vi "TTA_MATLAB_TxOutputPowerTest.vi"(0 "Sub-Function Name":string, 1 "Instrument Cluster In":T2, 5 "Test Group":string, 11 "error in":errorcluster) -> (4 "SubTestSuccess":dbl[](array[numeric]), 12 "Instrument Cluster Out":T2, 15 "error out":errorcluster)   [LabVIEW 2016]
uses:
  TTA_Controls/TTA_Control_Complete_Settings_Cluster.ctl
  TTA_Controls/TTA_Control_Instrument_Cluster.ctl
  TTA_Globals/TTA_Global_Complete_Settings.vi
panel:
  out "Tx Output \nPower Results":T1(array[cluster])
  out "Channel":string
  out "Tx":string
  out "Test Status":string
  in  "Complete Settings Cluster":T3
  out "RFICs":i32[](array[numeric])
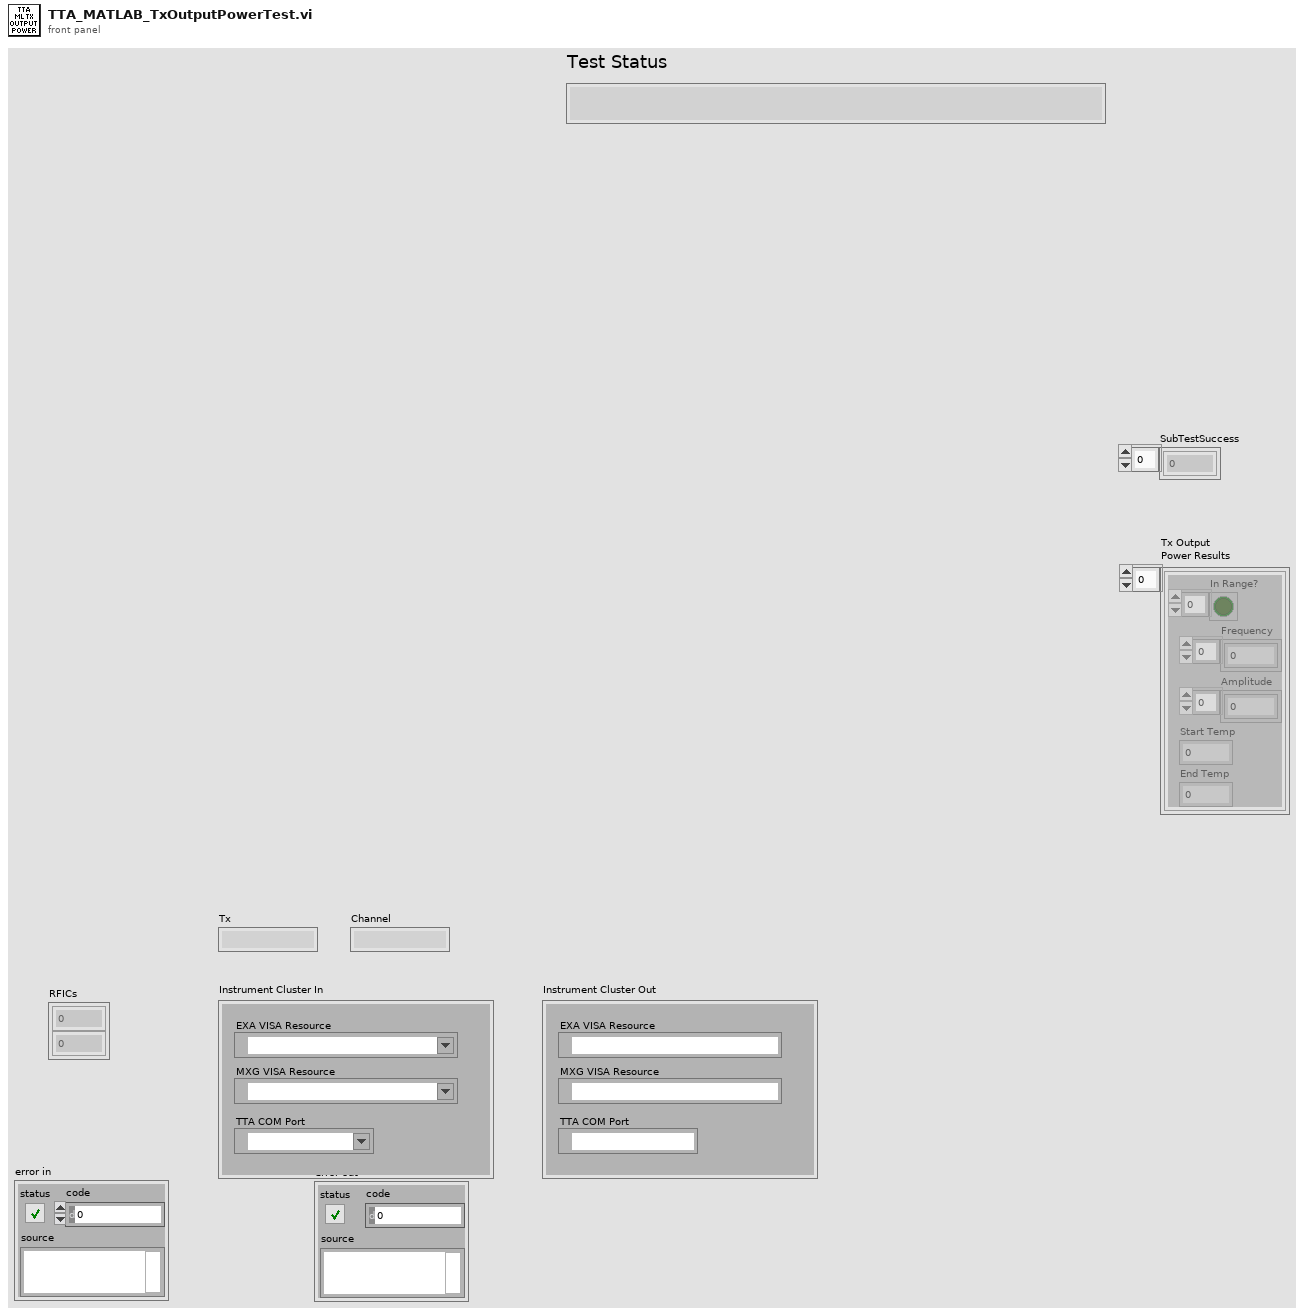
[diagram p1: front panel]
types:
  T1 = cluster{"In Range?":bool[], "Frequency":dbl[], "Amplitude":dbl[], "Start Temp":dbl, "End Temp":dbl}[]
  T2 = typedef "TTA_Control_Instrument_Cluster.ctl" = cluster{"EXA VISA Resource":refnum<visa-resource-name>, "MXG VISA Resource":refnum<visa-resource-name>, "TTA COM Port":refnum<visa-resource-name>}
  T3 = typedef "TTA_Control_Complete_Settings_Cluster.ctl" = cluster{"Brief Cluster":cluster{"STM Firmware File":string, "STM Firmware Address":string, "Required SW Version":string, "Template Used":string}, "Instrument Setting Cluster":cluster{"BDSFreq":dbl, "BDS Amp":dbl, "TxRFCal_Freq":dbl, "TxRFCal_Amp":dbl, "RxRFCal_Freq":dbl, "RxRFCal_Freq":dbl, "TxIF_Freq":dbl, "TxIF_Amp":dbl, "Tx_Output_Power_Signal_Freq":dbl, "Tx_ACPR_Signal_Freq":dbl, "Rx_RF_Freq":dbl, "Rx_RF_Amp":dbl, "Rx_Output_Power_Signal_Freq":dbl, "Rx_Output_Power_Sense_Freq":dbl}, "PAL Calibration\nInputs Cluster":cluster{"Amplitude Range\nMax(dBm)":dbl, "Amplitude Range\nMin(dBm)":dbl, "Amplitude Least\nCriteria (dBm)":dbl, "Frequency 1":dbl, "Frequency 2":dbl, "Frequency 3":dbl, "CAL Amplitude\nDecrement (dB)":dbl, "CAL Amplitude\nIncrement(dB)":dbl, "DownloadFile":string}, "TxOffset Cal Cluster":cluster{"Tx1 Offset (dB)":dbl, "Tx2 Offset (dB)":dbl, "Tx3 Offset (dB)":dbl, "Tx4 Offset (dB)":dbl, "Total RF Tx Loss (dB)":dbl}, "RxOffset Cal Cluster":cluster{"Rx1 Offset (dB)":dbl, "Rx2 Offset (dB)":dbl, "Rx3 Offset (dB)":dbl, "Rx4 Offset (dB)":dbl, "Total RF Rx Loss (dB)":dbl}, "TX Output Power Settings Cluster":cluster{"Frequency Sweep (MHz)":dbl[], "Sig Gen \nPower (dBm)":dbl, "Span (kHz)":dbl, "RBW (Hz)":dbl, "Ref Level (dBm)":dbl, "Low Power \nLimit":dbl, "High Power \nLimit":dbl, "DigAtt Max":dbl, "DigAtt Min":dbl}, "Tx ACPR Settings Cluster":cluster{"ACPR Filename":string, "Sampling Rate":dbl, "Power (dBm)":dbl, "IF Frequency Sweep (MHz)":dbl[], "State Name":string, "Mechanical\nAttenuation":dbl, "RefLevel Offset":dbl, "Amplitude Range\nMax (dBm)":dbl, "Amplitude Range\nMin (dBm)":dbl, "Cal Amp \nIncrement (dB)":dbl, "Cal Amp\nDecrement (dB)":dbl}, "Power Cal Cluster":cluster{"Power List (dBm)":dbl[], "Frequency (MHz)":dbl[], "Cal Decrement (dB)":dbl, "Cal Increment (dB)":dbl}, "Rx Received Power Settings Cluster":cluster{"Frequency Sweep (MHz)":dbl[], "Power (dBm)":dbl, "Span (kHz)":dbl, "RBW (Hz)":dbl, "Ref Level":dbl, "Low Power \nLimit (dBm)":dbl, "High Power\nLimit (dBm)":dbl}, "Tx Output Power Criteria Cluster":cluster{"CH1-TX1 \nMin":dbl, "CH1-TX1\nMax":dbl, "CH1-TXx3\nMin ":dbl, "CH1-TXx3\nMax":dbl, "CH2-TX1\nMin":dbl, "CH2-TX1\nMax":dbl, "CH2-TXx3\nMin":dbl, "CH2-TXx3\nMax":dbl}, "Tx ACPR Criteria Cluster":cluster{"Min Inband":dbl, "Max Close Outband":dbl, "Max Far Outband":dbl}, "Rx Output Power Criteria Cluster":cluster{"CH1-RX1 \nMin":dbl, "CH1-RX1 \nMax":dbl, "CH1-RXx3 \nMin":dbl, "CH1-RXx3\nMax":dbl, "CH2-RX1\nMin":dbl, "CH2-RX1\nMax":dbl, "CH2-RXx3\nMin":dbl, "CH2-RXx3\nMax":dbl}}
  T4 = cluster{"Amplitude Range\nMax(dBm)":dbl, "Amplitude Range\nMin(dBm)":dbl, "Amplitude Least\nCriteria (dBm)":dbl, "Frequency 1":dbl, "Frequency 2":dbl, "Frequency 3":dbl, "CAL Amplitude\nDecrement (dB)":dbl, "CAL Amplitude\nIncrement(dB)":dbl, "DownloadFile":string}
  T5 = cluster{"Frequency Sweep (MHz)":dbl[], "Sig Gen \nPower (dBm)":dbl, "Span (kHz)":dbl, "RBW (Hz)":dbl, "Ref Level (dBm)":dbl, "Low Power \nLimit":dbl, "High Power \nLimit":dbl, "DigAtt Max":dbl, "DigAtt Min":dbl}
  T6 = cluster{"In Range?":bool[], "Frequency":dbl[], "Amplitude":dbl[], "Start Temp":dbl, "End Temp":dbl}
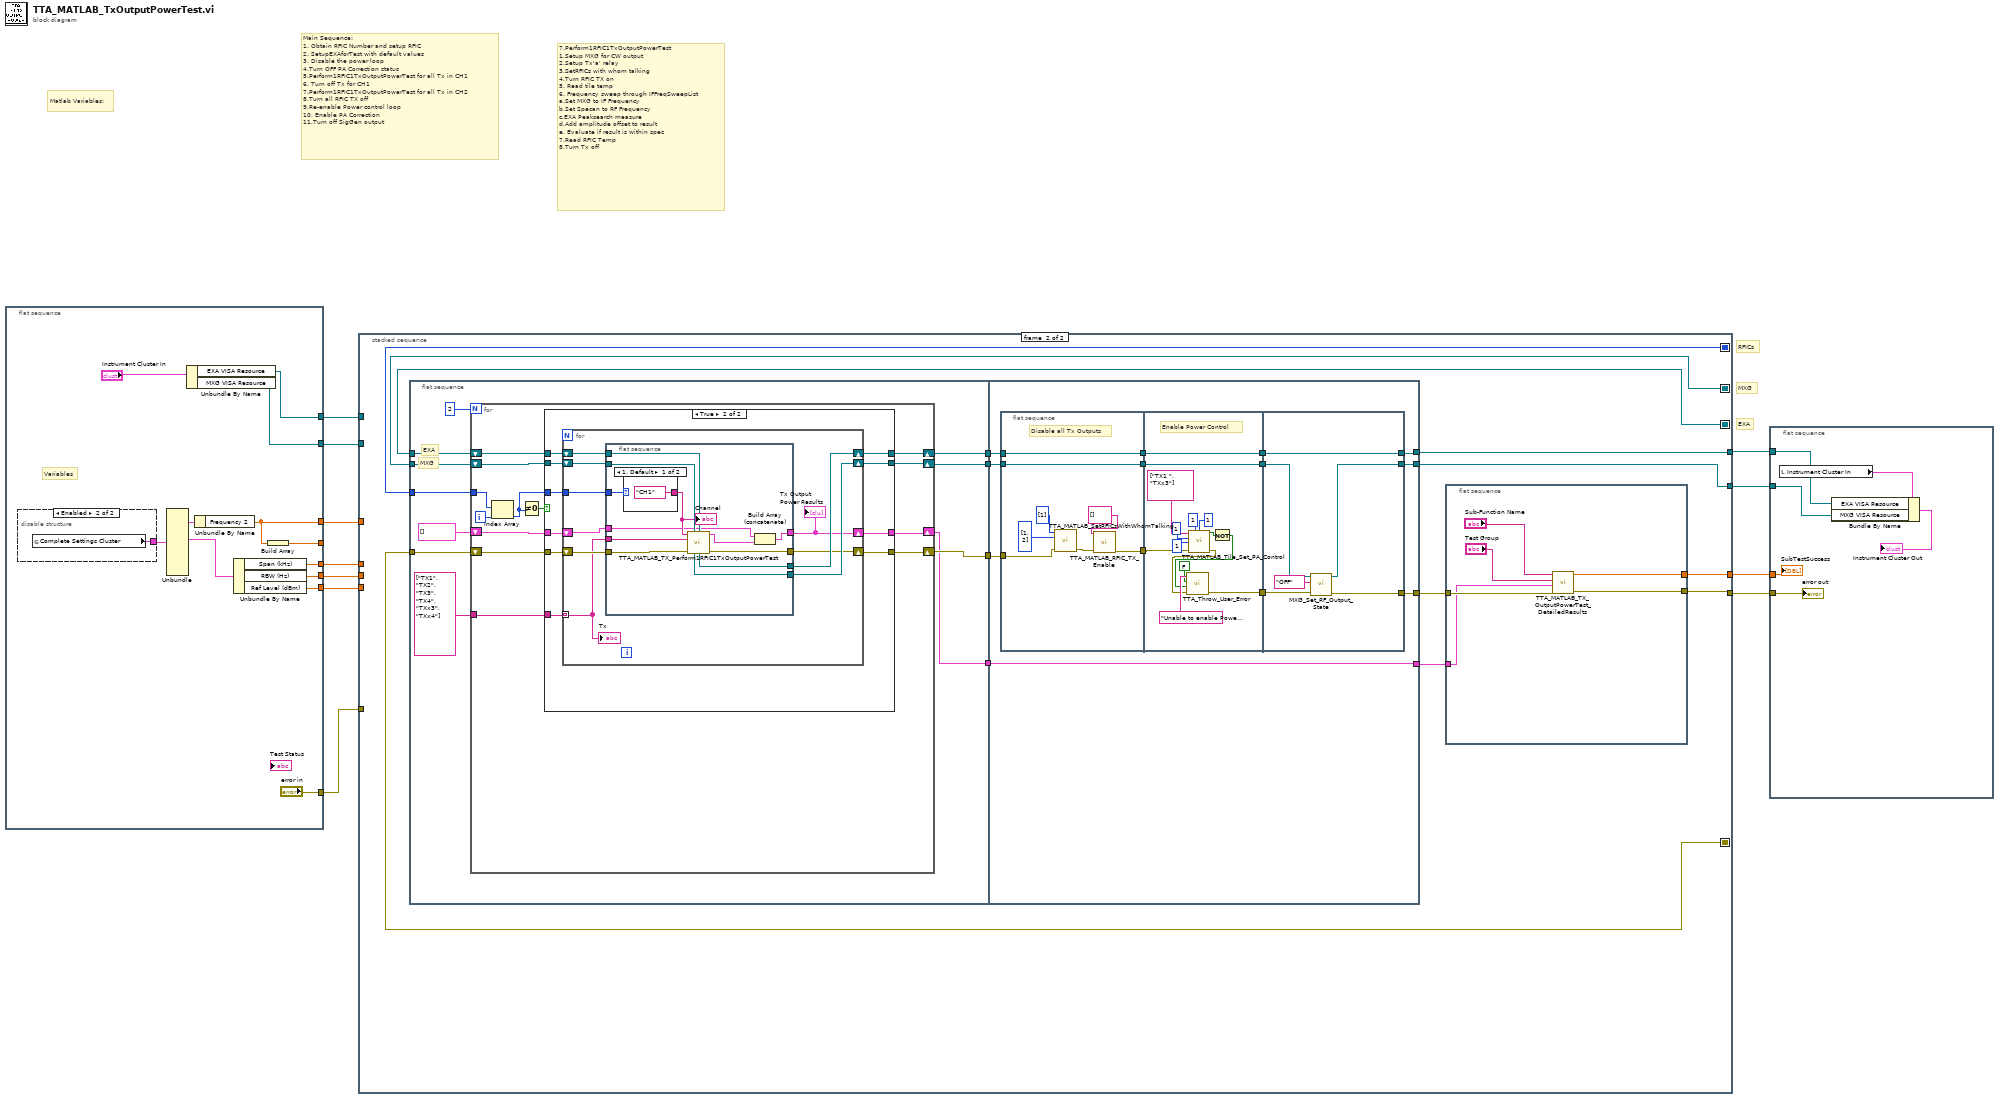
[diagram p0: block diagram]
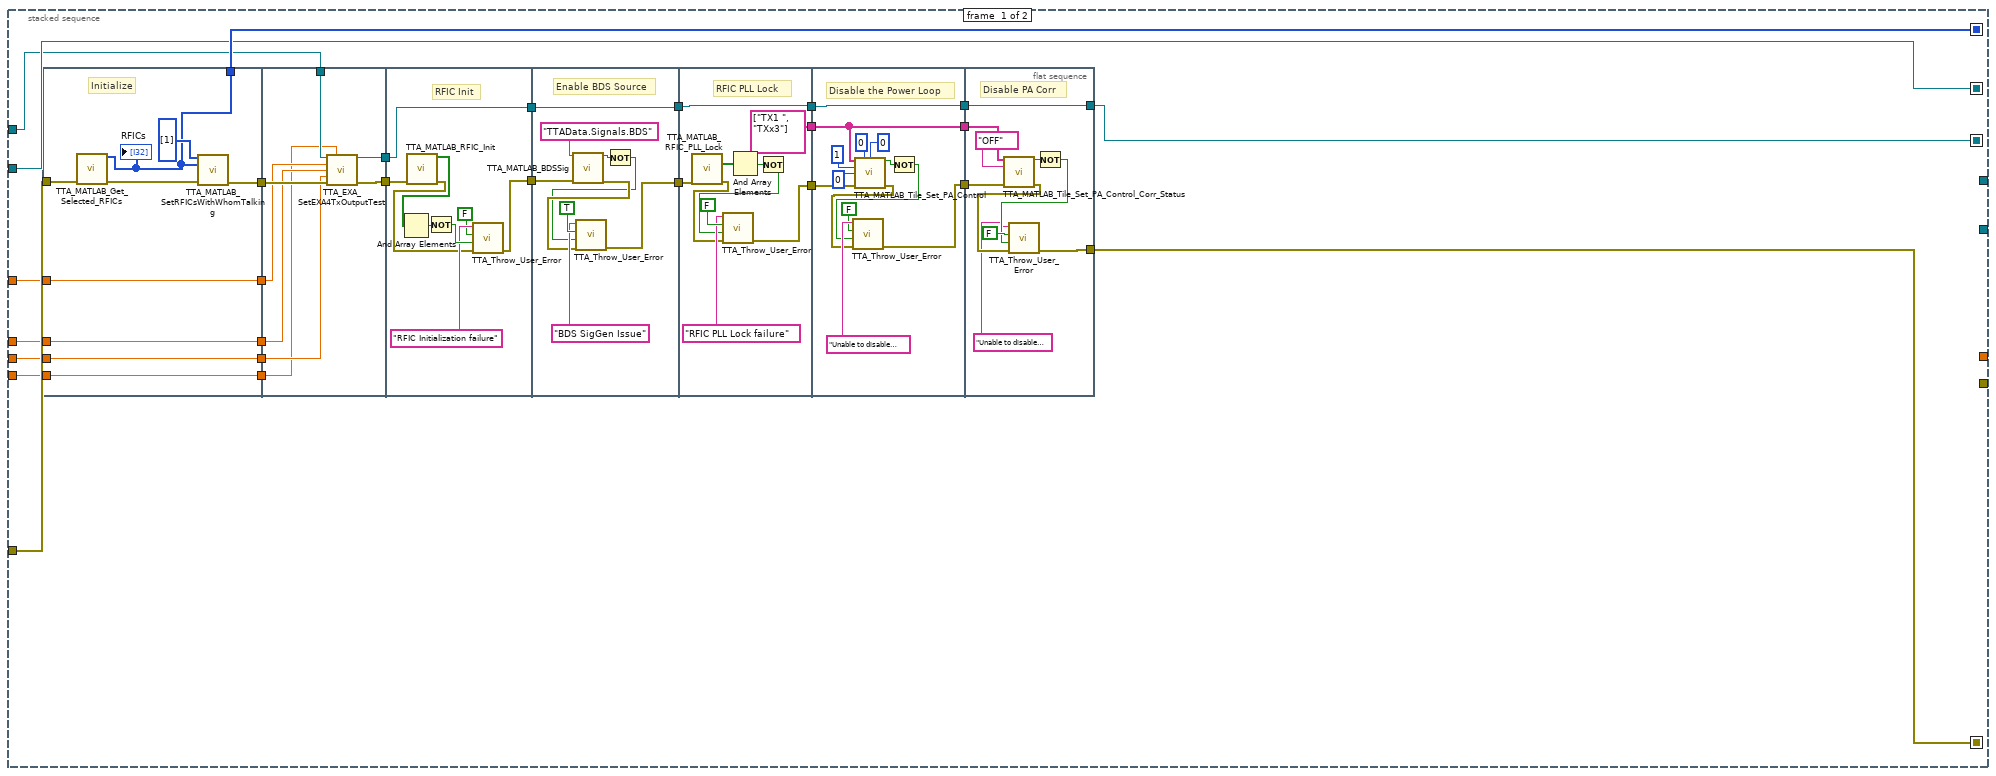
[diagram p2: hidden frame]
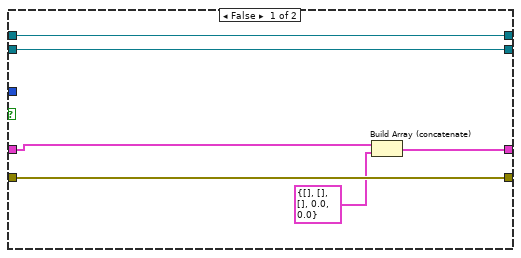
[diagram p3: hidden frame]
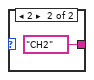
[diagram p4: hidden frame]
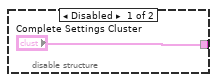
[diagram p5: hidden frame]
diagram:
  # "RFICs"
  # "EXA"
  # "MXG"
  # "Matlab Variables:"
  # "Main Sequence:\n1. Obtain RFIC Number and setup RFIC\n2. SetupEXAforTest with default values\n3. Disable the power loop\n4.Turn OFF PA Correction status\n5.Perform1RFIC1TxOutputPowerTest for all Tx in CH1\n6. Turn off Tx for CH1\n7.Perform1RFIC1TxOutputPowerTest for all Tx in CH2\n8.Turn all RFIC TX off\n9.Re-enable Power control loop\n10. Enable PA Correction\n11.Turn off SigGen output"
  # "7.Perform1RFIC1TxOutputPowerTest\n1.Setup MXG for CW output\n2.Setup Tx'a' relay\n3.SetRFICs with whom talking\n4.Turn RFIC TX on\n5. Read tile temp\n6. Frequency sweep through IFFreqSweepList\na.Set MXG to IF Frequency\nb.Set Specan to RF Frequency\nc.EXA Peaksearch measure\nd.Add amplitude offset to result\ne. Evaluate if result is within spec\n7.Read RFIC Temp\n8.Turn Tx off"
  n1 = flat-sequence {
    tunnel: ["error in"] -> w11
    tunnel: [w18] -> w10
    tunnel: [w17] -> w9
    tunnel: [w21] -> _
    tunnel: [w15] -> w5
    tunnel: [w14] -> w4
    tunnel: [w13] -> w3
    tunnel: [w12] -> w2
    frame #0 {
      # "Variables"
      n2 = disable-structure shown="Enabled" {
        disable-tunnel: ["Complete Settings Cluster" w25] -> w23
        frame Disabled {
        }
        frame Enabled {
          n3 = global read "TTA_Global_Complete_Settings.vi" "Complete Settings Cluster"() -> (w25:T3)
        }
      }
      n4 = Unbundle(w23) -> ("PAL Calibration\nInputs Cluster"=w20:T4, "TX Output Power Settings Cluster"=w16:T5)  [unwired: 10 out]
      n5 = Unbundle By Name("Instrument Cluster In") -> ("EXA VISA Resource"=w18:refnum<visa-resource-name>, "MXG VISA Resource"=w17:refnum<visa-resource-name>)
      n6 = Unbundle By Name(w20) -> ("Frequency 2"=w14:dbl)
      n7 = Unbundle By Name(w16) -> ("Span (kHz)"=w15:dbl, "RBW (Hz)"=w13:dbl, "Ref Level (dBm)"=w12:dbl)
      n8 = Build Array(w14) -> (w21:dbl[])
    }
  }
  n9 = stacked-sequence {
    seq-local: [w50 _] -> [_ w134]
    seq-local: [w28 _] -> [_ w132]
    seq-local: [w26 _] -> [_ w133]
    seq-local: [w44 _] -> [_ w131]
    tunnel: w11 -> [w52 _]
    tunnel: w10 -> [w37 _]
    tunnel: w9 -> [w44 _]
    tunnel: [_ w121] -> w8
    tunnel: [_ w127] -> w7
    tunnel: [_ w126] -> w6
    tunnel: w5 -> [w43 _]
    tunnel: w4 -> [w42 _]
    tunnel: w3 -> [w39 _]
    tunnel: w2 -> [w36 _]
    tunnel: [_ w122] -> w1
    frame #0 {
      n10 = flat-sequence {
        tunnel: w52 -> [w59]
        tunnel: [w58] -> w50
        tunnel: [w57] -> w49
        tunnel: w43 -> [w55]
        tunnel: w42 -> [w56]
        tunnel: [w56] -> w41
        tunnel: [w55] -> w40
        tunnel: w39 -> [w54]
        tunnel: [w54] -> w38
        tunnel: w36 -> [w53]
        tunnel: [w53] -> w35
        tunnel: w49 -> [w69]
        tunnel: [w63] -> w48
        tunnel: w41 -> [w68]
        tunnel: w40 -> [w67]
        tunnel: w38 -> [w66]
        tunnel: w37 -> [w65]
        tunnel: w35 -> [w64]
        tunnel: [w62] -> w34
        tunnel: w48 -> [w73]
        tunnel: [w71] -> w47
        tunnel: w34 -> [w70]
        tunnel: [w70] -> w33
        tunnel: w47 -> [w83]
        tunnel: [w81] -> w46
        tunnel: w33 -> [w79]
        tunnel: [w79] -> w32
        tunnel: [w94] -> w51
        tunnel: w46 -> [w91]
        tunnel: [string[] ["TX1 ", "TXx3"] ("Channels")] -> w45
        tunnel: w32 -> [w88]
        tunnel: [w88] -> w31
        tunnel: w51 -> [w106]
        tunnel: w45 -> [w99]
        tunnel: w31 -> [w98]
        tunnel: [w100] -> w30
        tunnel: [w99] -> w29
        tunnel: [w98] -> w27
        tunnel: w30 -> [w120]
        tunnel: w29 -> [w119]
        tunnel: [w112] -> w28
        tunnel: [w111] -> w26
        tunnel: w27 -> [w111]
        frame #0 {
          # "Initialize"
          n11 = call "TTA_MATLAB_Get_Selected_RFICs.vi"("error in"=w59) -> ("RFICs"=w58:i32[], "error out"=w60:errorcluster)  [unwired: 13 in]
          "RFICs" <- w58
          n12 = call "TTA_MATLAB_SetRFICsWithWhomTalking.vi"("Panel Array"=i32[] [1], "RFIC Array"=w58, "error in"=w60) -> ("error out"=w57:errorcluster)  [unwired: 12 in]
        }
        frame #1 {
          n13 = call "TTA_EXA_SetEXA4TxOutputTest.vi"("VISA resource In"=w65, "Reference Level (dBm)"=w64, "Frequency (MHz)"=w68, "Span (kHz)"=w67, "RBW (Hz)"=w66, "error in"=w69) -> ("VISA resource Out"=w62:refnum<visa-resource-name>, "error out"=w63:errorcluster)  [unwired: 8 in]
        }
        frame #2 {
          # "RFIC Init"
          n14 = call "TTA_MATLAB_RFIC_Init.vi"("error in"=w73) -> ("SuccessComm"=w78:bool[], "error out"=w72:errorcluster)  [unwired: 13 in]
          n15 = And Array Elements(Boolean array=w78) -> (logical AND=w77:bool)
          n16 = Not(x=w77) -> (.not. x?=w76:bool)
          n17 = call "TTA_Throw_User_Error.vi"("error in"=w72, "Error?"=w76, "Stop Execution on Fail"=FALSE, "Error Message"="RFIC Initialization failure") -> ("error out"=w71:errorcluster)  [unwired: 7 in]
        }
        frame #3 {
          # "Enable BDS Source"
          n18 = call "TTA_MATLAB_BDSSig.vi"("Signal Settings"="TTAData.Signals.BDS", "error in"=w83) -> ("Success"=w84:bool, "error out"=w82:errorcluster)  [unwired: 12 in]
          n19 = Not(x=w84) -> (.not. x?=w80:bool)
          n20 = call "TTA_Throw_User_Error.vi"("error in"=w82, "Error?"=w80, "Stop Execution on Fail"=TRUE, "Error Message"="BDS SigGen Issue") -> ("error out"=w81:errorcluster)  [unwired: 7 in]
        }
        frame #4 {
          # "RFIC PLL Lock"
          n21 = call "TTA_MATLAB_RFIC_PLL_Lock.vi"("error in"=w91) -> ("SuccessComm"=w97:bool[], "error out"=w90:errorcluster)  [unwired: 11 in, 2 out]
          n22 = And Array Elements(Boolean array=w97) -> (logical AND=w93:bool)
          n23 = Not(x=w93) -> (.not. x?=w92:bool)
          n24 = call "TTA_Throw_User_Error.vi"("error in"=w90, "Error?"=w92, "Stop Execution on Fail"=FALSE, "Error Message"="RFIC PLL Lock failure") -> ("error out"=w94:errorcluster)  [unwired: 7 in]
        }
        frame #5 {
          # "Disable the Power Loop"
          n25 = call "TTA_MATLAB_Tile_Set_PA_Control.vi"("Channels"=w99, "OutPower"=0, "InPower"=0, "Temp"=1, "Current"=0, "error in"=w106) -> ("Success"=w103:bool, "error out"=w101:errorcluster)  [unwired: 6 in, 2 out]
          n26 = Not(x=w103) -> (.not. x?=w102:bool)
          n27 = call "TTA_Throw_User_Error.vi"("error in"=w101, "Error?"=w102, "Stop Execution on Fail"=FALSE, "Error Message"="Unable to disable Power Loop") -> ("error out"=w100:errorcluster)  [unwired: 7 in]
        }
        frame #6 {
          # "Disable PA Corr"
          n28 = call "TTA_MATLAB_Tile_Set_PA_Control_Corr_Status.vi"("Channels"=w119, "ModeAdapt"="OFF", "error in"=w120) -> ("Success"=w116:bool, "error out"=w114:errorcluster)  [unwired: 9 in, 2 out]
          n29 = Not(x=w116) -> (.not. x?=w115:bool)
          n30 = call "TTA_Throw_User_Error.vi"("error in"=w114, "Error?"=w115, "Stop Execution on Fail"=FALSE, "Error Message"="Unable to disable PAL correction") -> ("error out"=w112:errorcluster)  [unwired: 7 in]
        }
      }
    }
    frame #1 {
      n31 = flat-sequence {
        tunnel: w134 -> [w151]
        tunnel: w133 -> [w150]
        tunnel: w131 -> [w149]
        tunnel: w132 -> [w148]
        tunnel: [w147] -> w130
        tunnel: [w146] -> w129
        tunnel: [w145] -> w128
        tunnel: [w142] -> w125
        tunnel: w130 -> [w217]
        tunnel: w129 -> [w216]
        tunnel: w128 -> [w215]
        tunnel: [w208] -> w123
        tunnel: [w207] -> w127
        tunnel: [w206] -> w126
        tunnel: w125 -> [w205]
        tunnel: [w205] -> w124
        frame #0 {
          # "EXA"
          # "MXG"
          n32 = for {
            N: 2 -> [_]
            tunnel: w151 -> [w154]
            shift-right: [w162] -> w146
            shift-left: w150 -> [w161]
            shift-right: [w159] -> w145
            shift-left: w149 -> [w160]
            shift-right: [w158] -> w147
            shift-left: w148 -> [w164]
            tunnel: string[] ["TX1", "TX2", "TX3", "TX4", "TXx3", "TXx4"] -> [w163]
            shift-right: [w156] -> w142
            shift-left: T1 [] -> [w157]
            i -> [w153]
            n33 = Index Array(array=w154, index=w153) -> (element=w152:i32)
            n34 = Not Equal To 0?(x=w152) -> (x != 0?=w155:bool)
            n35 = case shown="True" w155 {
              tunnel: w152 -> [_ w180]
              tunnel: w164 -> [w170 w179]
              tunnel: w163 -> [_ w178]
              tunnel: [w168 w177] -> w162
              tunnel: w161 -> [w168 w176]
              tunnel: w160 -> [w167 w175]
              tunnel: [w167 w174] -> w159
              tunnel: [w170 w173] -> w158
              tunnel: w157 -> [w166 w172]
              tunnel: [w169 w171] -> w156
              frame False {
                n36 = Build Array (concatenate)(w166, T6 {"In Range?"=[], "Frequency"=[], "Amplitude"=[], "Start Temp"=0.0, "End Temp"=0.0} ("Output Power\nResults")) -> (w169:T1)
              }
              frame True {
                n37 = for {
                  tunnel: w180 -> [w190]
                  tunnel: w178 -> [w188] mode=indexing
                  shift-right: [w187] -> w177
                  shift-left: w176 -> [w186]
                  shift-right: [w185] -> w174
                  shift-left: w175 -> [w184]
                  shift-right: [w183] -> w173
                  shift-left: w179 -> [w189]
                  shift-right: [w181] -> w171
                  shift-left: w172 -> [w182]
                  n38 = flat-sequence {
                    tunnel: w190 -> [w202]
                    tunnel: w186 -> [w201]
                    tunnel: w184 -> [w200]
                    tunnel: w189 -> [w199]
                    tunnel: w188 -> [w197]
                    tunnel: [w196] -> w187
                    tunnel: [w195] -> w185
                    tunnel: [w194] -> w183
                    tunnel: [w192] -> w181
                    tunnel: w182 -> [w191]
                    frame #0 {
                      n39 = case shown="1, Default" w202 {
                        tunnel: ["CH1" ("Channel") "CH2" ("Channel")] -> w198
                        frame 1, Default {
                        }
                        frame 2 {
                        }
                      }
                      "Channel" <- w198
                      n40 = call "TTA_MATLAB_TX_Perform1RFIC1TxOutputPowerTest.vi"("Channel"=w198, "MXG VISA Resource In"=w200, "EXA VISA Resource"=w201, "Tx"=w197, "error in"=w199) -> ("Output Power\nResults"=w193:T6, "MXG VISA Resource Out"=w195:refnum<visa-resource-name>, "EXA VISA Resource Out"=w196:refnum<visa-resource-name>, "error out"=w194:errorcluster)  [unwired: 7 in]
                      n41 = Build Array (concatenate)(w191, w193) -> (w192:T1)
                    }
                  }
                  "Tx" <- w188
                  "Tx Output \nPower Results" <- w181
                }
              }
            }
          }
        }
        frame #1 {
          n42 = flat-sequence {
            tunnel: w217 -> [w223]
            tunnel: w216 -> [w219]
            tunnel: w215 -> [w218]
            tunnel: [w220] -> w214
            tunnel: [w219] -> w213
            tunnel: [w218] -> w212
            tunnel: w214 -> [w228]
            tunnel: w213 -> [w239]
            tunnel: w212 -> [w238]
            tunnel: [w239] -> w211
            tunnel: [w238] -> w210
            tunnel: [w226] -> w209
            tunnel: [w242] -> w207
            tunnel: [w245] -> w206
            tunnel: w211 -> [w245]
            tunnel: w210 -> [w243]
            tunnel: w209 -> [w244]
            tunnel: [w240] -> w208
            frame #0 {
              # "Disable all Tx Outputs"
              n43 = call "TTA_MATLAB_SetRFICsWithWhomTalking.vi"("Panel Array"=i32[] [1], "RFIC Array"=i32[] [1, 2], "error in"=w223) -> ("error out"=w221:errorcluster)  [unwired: 12 in]
              n44 = call "TTA_MATLAB_RFIC_TX_Enable.vi"("Channels"=string[] [], "error in"=w221) -> ("error out"=w220:errorcluster)  [unwired: 12 in, 1 out]
            }
            frame #1 {
              # "Enable Power Control"
              n45 = call "TTA_MATLAB_Tile_Set_PA_Control.vi"("Channels"=string[] ["TX1 ", "TXx3"], "OutPower"=1, "InPower"=1, "Temp"=1, "Current"=1, "error in"=w228) -> ("Success"=w231:bool, "error out"=w229:errorcluster)  [unwired: 6 in, 2 out]
              n46 = Not(x=w231) -> (.not. x?=w230:bool)
              n47 = call "TTA_Throw_User_Error.vi"("error in"=w229, "Error?"=w230, "Stop Execution on Fail"=FALSE, "Error Message"="Unable to enable Power Loop") -> ("error out"=w226:errorcluster)  [unwired: 7 in]
            }
            frame #2 {
              n48 = call "MXG_Set_RF_Output_State.vi"("error in"=w244, "RF Output State"="OFF", "VISA resource name"=w243) -> ("error out"=w240:errorcluster, "VISA resource name"=w242:refnum<visa-resource-name>)  [unwired: 7 in]
            }
          }
        }
      }
      n49 = flat-sequence {
        tunnel: w124 -> [w137]
        tunnel: w123 -> [w140]
        tunnel: [w136] -> w122
        tunnel: [w135] -> w121
        frame #0 {
          n50 = call "TTA_MATLAB_TX_OutputPowerTest_DetailedResults.vi"("error in"=w140, "Tx Output \nPower Results"=w137, "TestGroup"="Test Group", "SubTest"="Sub-Function Name") -> ("error out"=w135:errorcluster, "SubTestSuccess"=w136:dbl[])  [unwired: 6 in]
        }
      }
    }
  }
  n51 = flat-sequence {
    tunnel: w8 -> [w251]
    tunnel: w7 -> [w248]
    tunnel: w6 -> [w249]
    tunnel: w1 -> [w246]
    frame #0 {
      n52 = local read "Instrument Cluster In"() -> (w247:T2)
      n53 = Bundle By Name(cluster=w247, "EXA VISA Resource"=w249, "MXG VISA Resource"=w248) -> (→"Instrument Cluster Out":T2)
      "error out" <- w251
      "SubTestSuccess" <- w246
    }
  }
